vi "Create Template Layer.vi"(10 "Lib Color":u32, 11 "Project Name":string) -> (1 "Color Image":T1, 2 "new picture":picture, 3 "Icon out":refnum<class "Icon.lvclass">)   [LabVIEW 2021, in "Plugin Generator.lvlib"]
uses:
  Plugin Generator.lvlib
  <vilib>/LabVIEW Icon API/lv_icon/Classes/Icon/Icon.lvclass
  <vilib>/picture/picture.llb/imagedata.ctl
  <vilib>/LabVIEW Icon API/API_Test Settings.ctl
  <vilib>/LabVIEW Icon API/lv_icon/Controls/Alignment.ctl
  <vilib>/LabVIEW Icon API/API_Text Colors.ctl
  <vilib>/LabVIEW Icon API/API_Text.ctl
  <vilib>/LabVIEW Icon API/API_Rectangle Dimension.ctl
  <vilib>/LabVIEW Icon API/API_Rectangle Colors.ctl
  <vilib>/LabVIEW Icon API/LabVIEW Icon API.lvlib
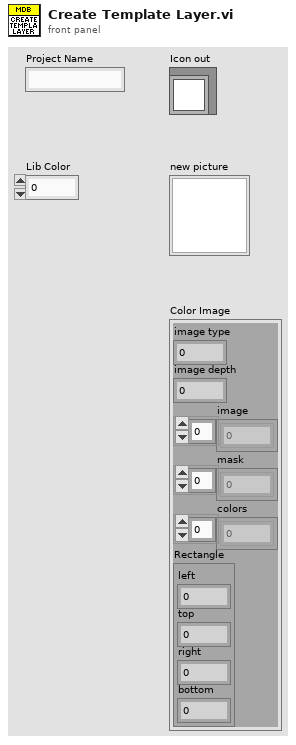
[diagram p1: front panel]
types:
  T1 = typedef "imagedata.ctl" = cluster{"image type":i32, "image depth":i32, "image":u8[], "mask":u8[], "colors":u32[], "Rectangle":cluster{"left":i16, "top":i16, "right":i16, "bottom":i16}}
  T2 = typedef "LabVIEW Icon API.lvlib/API_Rectangle Colors.ctl" = cluster{"Border":u32, "Background":u32}
  T3 = typedef "LabVIEW Icon API.lvlib/API_Rectangle Dimension.ctl" = cluster{"Width":i16, "Height":i16}
  T4 = typedef "LabVIEW Icon API.lvlib/API_Text.ctl" = cluster{"Line 1 text":string, "Line 2 text":string, "Line 3 text":string, "Line 4 text":string}
  T5 = typedef "LabVIEW Icon API.lvlib/API_Test Settings.ctl" = cluster{"Font":string, "Alignment":T6, "Size":u8, "Center text":bool, "Capitalize text":bool, "Text color":T7}
  T6 = typedef "Alignment.ctl" = u16
  T7 = typedef "LabVIEW Icon API.lvlib/API_Text Colors.ctl" = cluster{"Line 1 color":u32, "Line 2 color":u32, "Line 3 color":u32, "Line 4 color":u32}
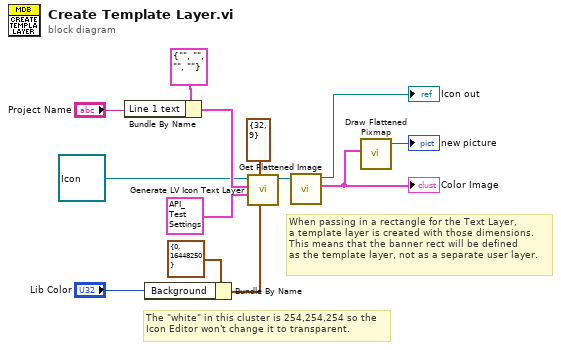
[diagram p0: block diagram]
diagram:
  # "The \"white\" in this cluster is 254,254,254 so the\nIcon Editor won't change it to transparent."
  # "When passing in a rectangle for the Text Layer,\na template layer is created with those dimensions.\nThis means that the banner rect will be defined\nas the template layer, not as a separate user layer."
  n1 = Bundle By Name(cluster=T4 {"Line 1 text"="", "Line 2 text"="", "Line 3 text"="", "Line 4 text"=""} ("Text"), "Line 1 text"="Project Name") -> (w6:T4)
  n2 = Bundle By Name(cluster=T2 {"Border"=0, "Background"=16448250} ("Rectangle colors (black, white)"), "Background"="Lib Color") -> (w12:T2)
  n3 = call <vilib>:"Generate LV Icon Text Layer.vi"("Rectangle colors (black, white)"=w12, "Rectangle dimension (32,32)"=T3 {"Width"=32, "Height"=9}, "Text settings"=T5 {"Font"="Small Fonts", "Alignment"=1, "Size"=8, "Center text"=TRUE, "Capitalize text"=TRUE, "Text color"={"Line 1 color"=0, "Line 2 color"=0, "Line 3 color"=0, "Line 4 color"=0}}, "Text"=w6, "Icon in"=refnum<class "Icon.lvclass"> refnum ("Icon.lvclass in")) -> ("Icon out"=w2:refnum<class "Icon.lvclass">)  [unwired: 5 in, 1 out]
  n4 = call <vilib>:"Get Flattened Image.vi"("lv_icon.lvlib:Icon.lvclass in"=w2) -> ("Color Image"=w8:T1, "lv_icon.lvlib:Icon.lvclass out"=→"Icon out":refnum<class "Icon.lvclass">)  [unwired: 7 in, 2 out]
  "Color Image" <- w8
  n5 = call <vilib>:"Draw Flattened Pixmap.vi"("image data"=w8) -> ("new picture"=→"new picture":picture)  [unwired: 8 in]
